vi "CU_WriteSolutionToStr.vi"(7 "ListBox Ref in":refnum<vi>, 8 "Solution in":string[](array[string]), 9 "Iteration Num":i32, 10 "Dataset Num":i32, 11 "String Ref in":refnum<vi>) -> (0 "error out":errorcluster, 3 "String out":string)   [LabVIEW 2016, in "Classifier.lvlib"]
uses:
  Classifier.lvlib
panel:
  # "This VI is a part of BCI Design library, http://www.ru-bci.org \nCopyright © 2020, Sotnikov Peter, All rights reserved. License: GNU GPLv3"
  # "Поколение"
  # "Точность\nна тестовой\nвыборке"
  # "Размерность\nвектора\nпризнаков"
  # "Точность\nна обучающей\nвыборке"
  # "Точность\nна контрол. \nвыборке"
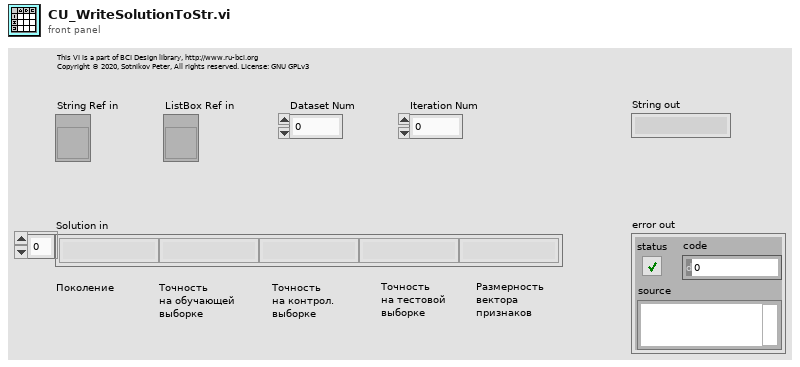
[diagram p1: front panel]
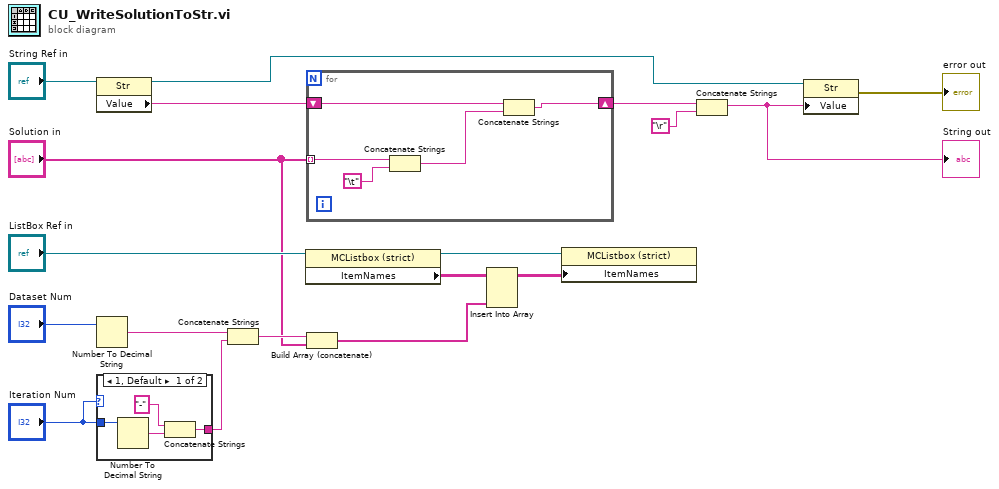
[diagram p0: block diagram]
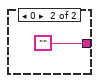
[diagram p2: hidden frame]
diagram:
  n1 = property class="Str"(reference="String Ref in") -> (reference out=w13:refnum<vi>, "Value"=w17:string)  [unwired: 1 in, 1 out]
  n2 = Number To Decimal String(number="Dataset Num") -> (decimal integer string=w10:string)  [unwired: 1 in]
  n3 = case shown="1, Default" "Iteration Num" {
    tunnel: "Iteration Num" -> [w22 _]
    tunnel: [w20 ""] -> w1
    frame 1, Default {
      n4 = Number To Decimal String(number=w22) -> (decimal integer string=w21:string)  [unwired: 1 in]
      n5 = Concatenate Strings("-" ("string"), w21) -> (w20:string)
    }
    frame 0 {
    }
  }
  n6 = Concatenate Strings(w10, w1) -> (w8:string)
  n7 = property class="MCListbox (strict)"(reference="ListBox Ref in") -> (reference out=w6:refnum<vi>, "ItemNames"=w5:string[][])  [unwired: 1 in, 1 out]
  n8 = for {
    shift-right: [w27] -> w16
    shift-left: w17 -> [w28]
    tunnel: "Solution in" -> [w25] mode=indexing
    n9 = Concatenate Strings(w25, "\t") -> (w24:string)
    n10 = Concatenate Strings(w28, w24) -> (w27:string)
  }
  n11 = Build Array (concatenate)(w8, "Solution in") -> (w3:string[])
  n12 = Insert Into Array(array=w5, new element=w3) -> (w4:string[][])  [unwired: 2 in]
  n13 = property class="MCListbox (strict)"(reference=w6, "ItemNames"=w4) -> ()  [unwired: 1 in, 2 out]
  n14 = Concatenate Strings(w16, "\r") -> (w14:string)
  "String out" <- w14
  n15 = property class="Str"(reference=w13, "Value"=w14) -> (error out=→"error out":errorcluster)  [unwired: 1 in, 1 out]
